vi "Write glide.vi"(8 "error in (no error)":errorcluster, 10 "glide":bool, 11 "Level in":refnum<class "Level.lvclass">) -> (0 "error out":errorcluster, 3 "Level out":refnum<class "Level.lvclass">)   [LabVIEW 2020, in "Level.lvclass"]
uses:
  Level.lvclass
  Level.lvclass/Level.ctl
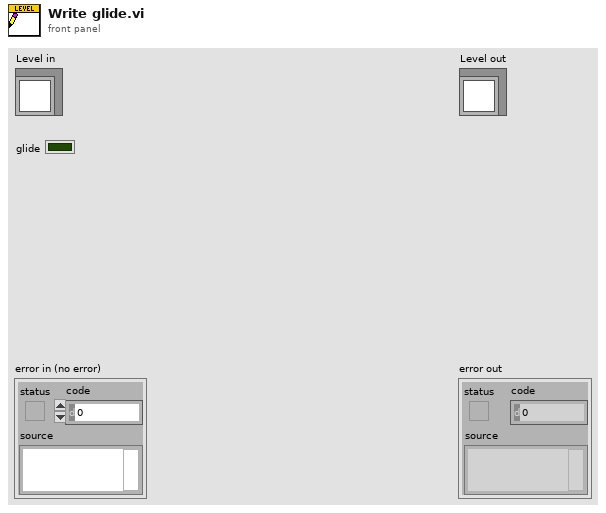
[diagram p1: front panel]
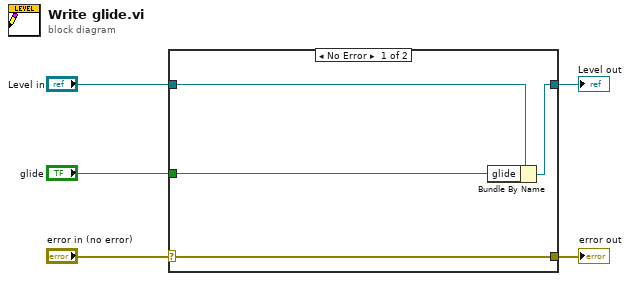
[diagram p0: block diagram]
diagram:
  n1 = case shown="No Error" "error in (no error)" {
    selector: "error in (no error)" -> [w9 w10]
    tunnel: [w9 w10] -> w4
    tunnel: [w7 w11] -> w2
    tunnel: "Level in" -> [w8 w11]
    tunnel: "glide" -> [w6 _]
    frame No Error {
      n2 = Bundle By Name(cluster=w8, "glide"=w6) -> (w7:refnum<class "Level.lvclass">)
    }
    frame Error {
    }
  }
  "error out" <- w4
  "Level out" <- w2
